vi "Stop App.vi"(8 "error in (no error)":errorcluster, 10 "activity name":string="com.team254.cheezdroid", 11 "AdbBridge in":refnum<class "Adb Bridge.lvclass">) -> (0 "error out":errorcluster, 3 "AdbBridge out":refnum<class "Adb Bridge.lvclass">)   [LabVIEW 2016, in "Adb Bridge.lvclass"]
uses:
  Adb Bridge.lvclass
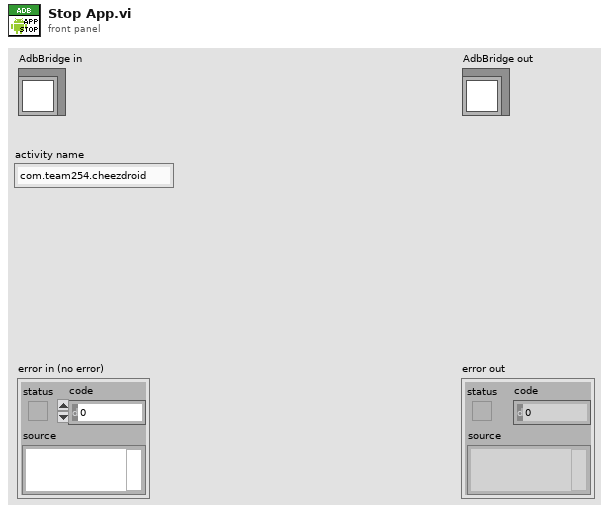
[diagram p1: front panel]
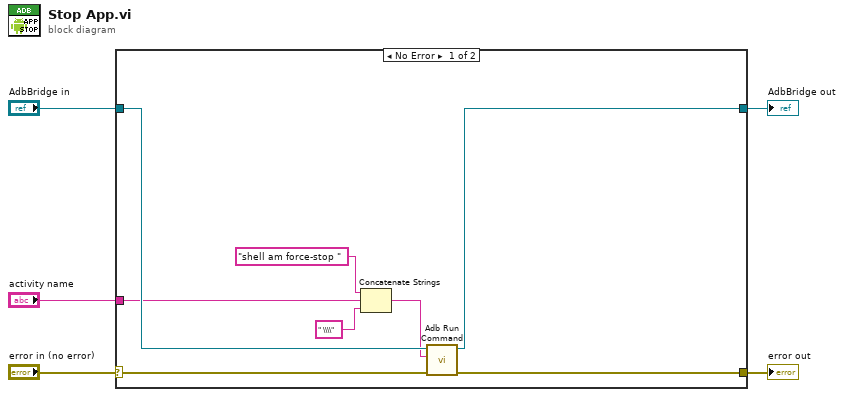
[diagram p0: block diagram]
diagram:
  n1 = case shown="No Error" "error in (no error)" {
    selector: "error in (no error)" -> [w12 w15]
    tunnel: [w11 w15] -> w4
    tunnel: [w10 w14] -> w2
    tunnel: "AdbBridge in" -> [w13 w14]
    tunnel: "activity name" -> [w9 _]
    frame No Error {
      n2 = Concatenate Strings("shell am force-stop " ("args"), w9, " \\\\" ("args")) -> (w6:string)
      n3 = call "Adb Run Command.vi"("error in (no error)"=w12, "args"=w6, "AdbBridge in"=w13) -> ("error out"=w11:errorcluster, "AdbBridge out"=w10:refnum<class "Adb Bridge.lvclass">)  [unwired: 7 in]
    }
    frame Error {
    }
  }
  "error out" <- w4
  "AdbBridge out" <- w2
